vi "QMH_UI_Control_EnQueue.vi"(7 "Last ?":bool, 8 "error in (no error)":errorcluster caption="entrée d'erreur (pas d'erreur)", 9 "Variant":variant, 10 "Command":T1=enum."UI Exit", 11 "UI Queue":refnum<queue>) -> (0 "error out":errorcluster caption="sortie d'erreur", 3 "UI Queue":refnum<queue>)   [LabVIEW 2020]
doc: "This VI enqueues an element to the QMH_UI queue, according to the input command, wich is the enum QMH_UI_Command.ctl."
uses:
  controls/QMH_UI_Message.ctl
  controls/QMH_UI_Command.ctl
panel:
  in  "QMH UI Message":T2
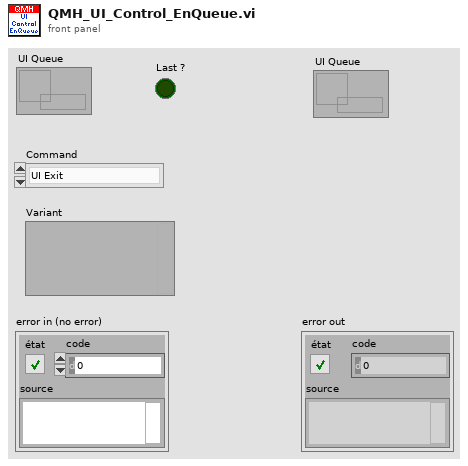
[diagram p1: front panel]
types:
  T1 = typedef "QMH_UI_Command.ctl" = enum16{"Initialize", "UI Load", "UI Save", "UI Save As", "UI Change Experiment", "UI Change Voltages", "UI Change Sequence", "UI Change Expert", "UI Change Loops", "UI Change Scientist", "Ready to Start", "UI Start", "Waiting for ICR", "UI Exit", "Update Report", "Update ICR Status", "Waiting for User"}
  T2 = typedef "QMH_UI_Message.ctl" = cluster{"Command":T1, "Data":variant}
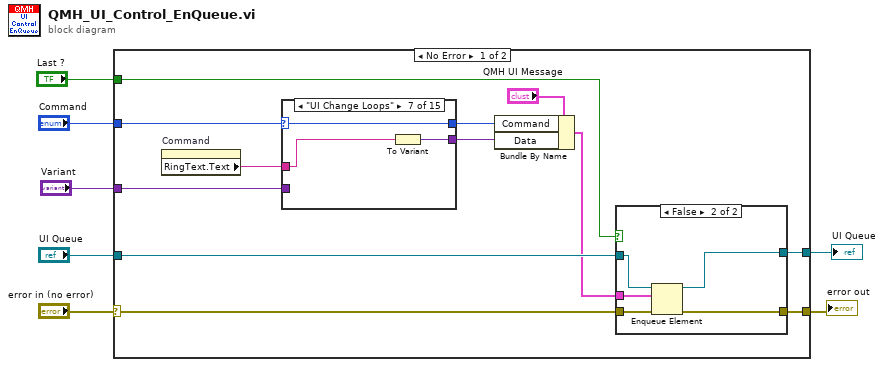
[diagram p0: block diagram]
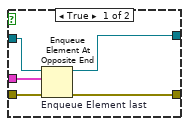
[diagram p2: hidden frame]
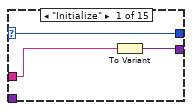
[diagram p3: hidden frame]
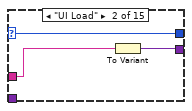
[diagram p4: hidden frame]
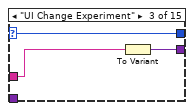
[diagram p5: hidden frame]
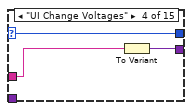
[diagram p6: hidden frame]
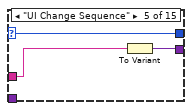
[diagram p7: hidden frame]
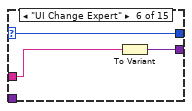
[diagram p8: hidden frame]
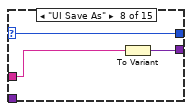
[diagram p9: hidden frame]
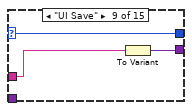
[diagram p10: hidden frame]
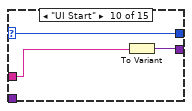
[diagram p11: hidden frame]
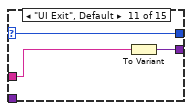
[diagram p12: hidden frame]
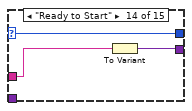
[diagram p15: hidden frame]
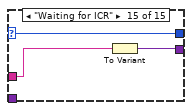
[diagram p16: hidden frame]
diagram:
  n1 = case shown="No Error" "error in (no error)" {
    selector: "error in (no error)" -> [w16 w73]
    tunnel: [w15 w73] -> w6
    tunnel: "UI Queue" -> [w18 _]
    tunnel: [w17 _] -> w4
    tunnel: "Command" -> [w14 _]
    tunnel: "Variant" -> [w12 _]
    tunnel: "Last ?" -> [w9 _]
    frame No Error {
      n2 = property on="Command" class="Enum (strict)"() -> ("RingText.Text"=w10:string)  [unwired: 2 in, 2 out]
      n3 = case shown="\"UI Change Loops\"" w14 {
        selector: w14 -> [w32 w35 w38 w41 w44 w47 w50 w53 w56 w59 w62 w64 w66 w69 w72]
        tunnel: [w31 w34 w36 w39 w43 w45 w48 w52 w55 w58 w61 w63 w65 w67 w70] -> w11
        tunnel: [w32 w35 w38 w41 w44 w47 w50 w53 w56 w59 w62 w64 w66 w69 w72] -> w13
        tunnel: w12 -> [_ _ _ _ _ _ _ _ _ _ _ w63 w65 _ _]
        tunnel: w10 -> [w30 w33 w37 w40 w42 w46 w49 w51 w54 w57 w60 _ _ w68 w71]
        frame "Initialize" {
          n4 = To Variant(anything=w30) -> (Variant=w31:variant)
        }
        frame "UI Load" {
          n5 = To Variant(anything=w33) -> (Variant=w34:variant)
        }
        frame "UI Change Experiment" {
          n6 = To Variant(anything=w37) -> (Variant=w36:variant)
        }
        frame "UI Change Voltages" {
          n7 = To Variant(anything=w40) -> (Variant=w39:variant)
        }
        frame "UI Change Sequence" {
          n8 = To Variant(anything=w42) -> (Variant=w43:variant)
        }
        frame "UI Change Expert" {
          n9 = To Variant(anything=w46) -> (Variant=w45:variant)
        }
        frame "UI Change Loops" {
          n10 = To Variant(anything=w49) -> (Variant=w48:variant)
        }
        frame "UI Save As" {
          n11 = To Variant(anything=w51) -> (Variant=w52:variant)
        }
        frame "UI Save" {
          n12 = To Variant(anything=w54) -> (Variant=w55:variant)
        }
        frame "UI Start" {
          n13 = To Variant(anything=w57) -> (Variant=w58:variant)
        }
        frame "UI Exit", Default {
          n14 = To Variant(anything=w60) -> (Variant=w61:variant)
        }
        frame "Update Report" {
        }
        frame "Update ICR Status" {
        }
        frame "Ready to Start" {
          n15 = To Variant(anything=w68) -> (Variant=w67:variant)
        }
        frame "Waiting for ICR" {
          n16 = To Variant(anything=w71) -> (Variant=w70:variant)
        }
      }
      n17 = Bundle By Name(cluster="QMH UI Message", "Command"=w13, "Data"=w11) -> (w8:T2)
      n18 = case shown="False" w9 {
        tunnel: w8 -> [w24 w29]
        tunnel: w18 -> [w23 w28]
        tunnel: [w22 w27] -> w17
        tunnel: w16 -> [w21 w26]
        tunnel: [w20 w25] -> w15
        frame True {
          n19 = Enqueue Element At Opposite End "Enqueue Element last"(queue=w23, element=w24, error in (no error)=w21) -> (queue out=w22:refnum<queue>, error out=w20:errorcluster)  [unwired: 1 in, 1 out]
        }
        frame False {
          n20 = Enqueue Element(queue=w28, element=w29, error in (no error)=w26) -> (queue out=w27:refnum<queue>, error out=w25:errorcluster)  [unwired: 2 out]
        }
      }
    }
    frame Error {
    }
  }
  "error out" <- w6
  "UI Queue" <- w4
